vi "LoadWaveShape.vi"(8 "error in":errorcluster) -> (0 "error out":errorcluster)   [LabVIEW 2018, in "AcPwrPlugins.lvlib" / "NHRGridSim.lvclass"]
uses:
  NHRGridSim.lvclass
panel:
  in  "State":enum16{"Initialize", "Events"}(ring)
  out "XY Graph":cluster{"X":dbl, "Y":dbl}[](graph)
  out "Q4":picture
  out "Q3":picture
  out "Q2":picture
  out "Q1":picture
  out "FileName":string
  in  "Load Button":bool
  out "Data":string
  out "Qx4":dbl[](array[numeric])
  out "Qx3":dbl[](array[numeric])
  out "Qx2":dbl[](array[numeric])
  out "Qx1":dbl[](array[numeric])
  out "Quad4":dbl[](array[numeric])
  out "Quad3":dbl[](array[numeric])
  out "Quad2":dbl[](array[numeric])
  out "Quad1":dbl[](array[numeric])
  in  "Cancel Button":bool
  in  "OK Button":bool
  in  "User":enum32{"User2", "User3", "User4"}(radio)
  # "Open the file containing the Wave Shape data to be loaded into the specified NHR \"USER\" AC instrument:"
  # "Load waveform to..."
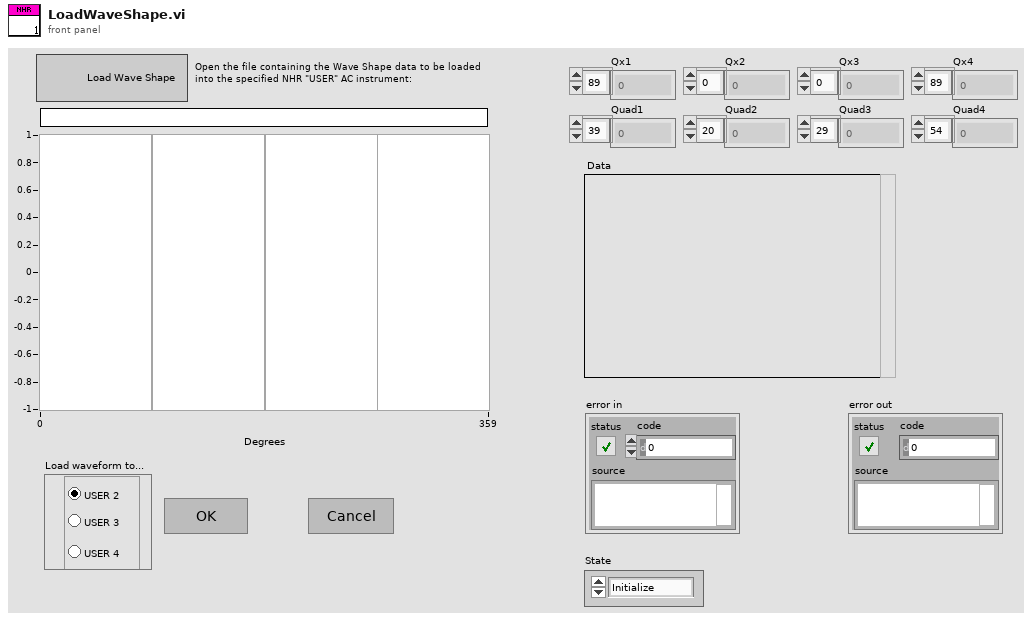
[diagram p1: front panel]
types:
  T1 = typedef "LVRectTypeDef.ctl" = cluster{"Left":i16, "Top":i16, "Right":i16, "Bottom":i16}
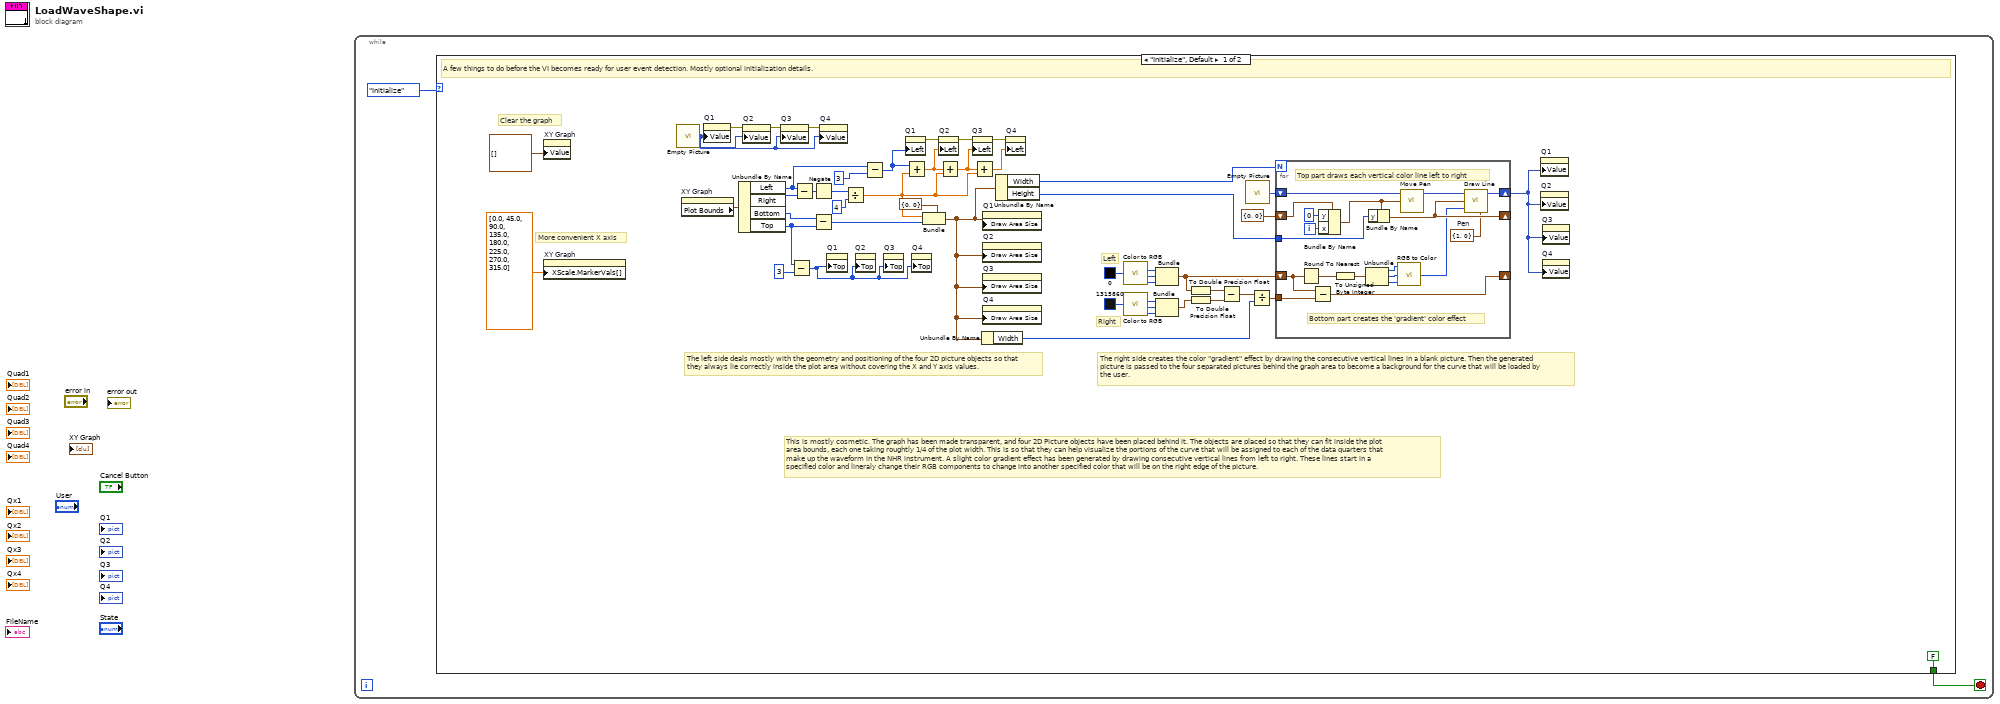
[diagram p0: block diagram]
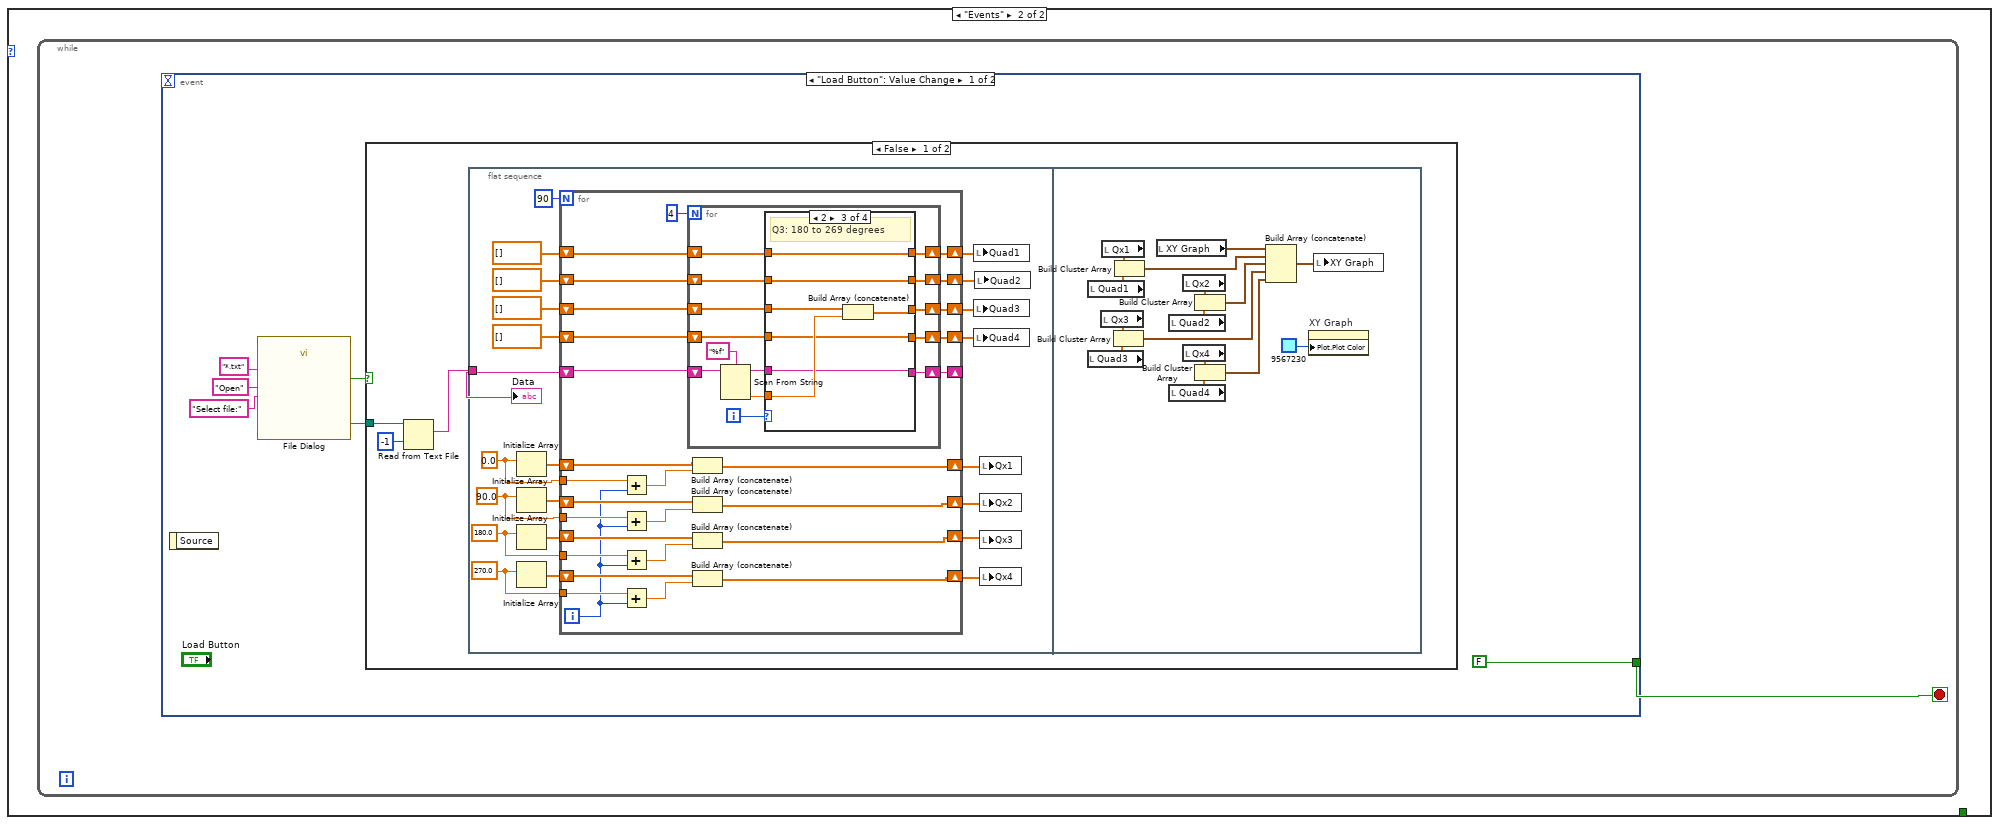
[diagram p2: hidden frame]
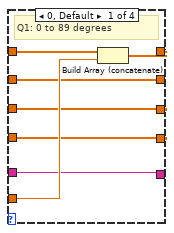
[diagram p3: hidden frame]
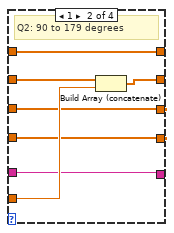
[diagram p4: hidden frame]
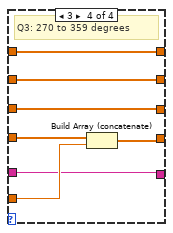
[diagram p5: hidden frame]
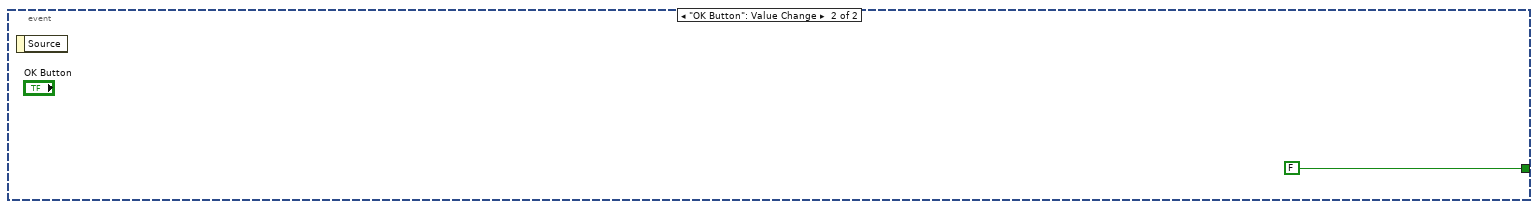
[diagram p7: hidden frame]
diagram:
  n1 = while {
    stop <- w1 stop-if-true
    n2 = case shown="\"Initialize\", Default" enum16{"Initialize", "Events"}."Initialize" ("State") {
      tunnel: [FALSE _] -> w1
      frame "Initialize", Default {
        # "The right side creates the color \"gradient\" effect by drawing the consecutive vertical lines in a blank picture. Then the generated picture is passed to the four separated pictures behind the graph area to become a background for the curve that will be loaded by the user."
        # "The left side deals mostly with the geometry and positioning of the four 2D picture objects so that they always lie correctly inside the plot area without covering the X and Y axis values."
        # "This is mostly cosmetic. The graph has been made transparent, and four 2D Picture objects have been placed behind it. The objects are placed so that they can fit inside the plot area bounds, each one taking roughtly 1/4 of the plot width. This is so that they can help visualize the portions of the curve that will be assigned to each of the data quarters that make up the waveform in the NHR instrument. A slight color gradient effect has been generated by drawing consecutive vertical lines from left to right. These lines start in a specified color and lineraly change their RGB components to change into another specified color that will be on the right edge of the picture."
        # "Right"
        # "Left"
        # "Clear the graph"
        # "More convenient X axis"
        # "A few things to do before the VI becomes ready for user event detection. Mostly optional initialization details."
        n3 = property on="XY Graph" class="XYGraph (strict)"("Value"=cluster{"element":dbl, dbl}[] [] ("array of clusters")) -> ()  [unwired: 2 in, 2 out]
        n4 = property on="XY Graph" class="XYGraph (strict)"("XScale.MarkerVals[]"=dbl[] [0.0, 45.0, 90.0, 135.0, 180.0, 225.0, 270.0, 315.0] ("X Scale.Marker Values[]")) -> ()  [unwired: 2 in, 2 out]
        n5 = call "Empty Picture"() -> ("empty picture"=w27:picture)
        n6 = property on="XY Graph" class="XYGraph (strict)"() -> ("Plot Bounds"=w28:T1)  [unwired: 2 in, 2 out]
        n7 = property on="Q1" class="Pict"("Value"=w27) -> (error out=w24:errorcluster)  [unwired: 2 in, 1 out]
        n8 = Unbundle By Name(w28) -> ("Left"=w45:i16, "Right"=w36:i16, "Bottom"=w48:i16, "Top"=w49:i16)
        n9 = property on="Q2" class="Pict"(error in=w24, "Value"=w27) -> (error out=w25:errorcluster)  [unwired: 1 in, 1 out]
        n10 = property on="Q3" class="Pict"(error in=w25, "Value"=w27) -> (error out=w26:errorcluster)  [unwired: 1 in, 1 out]
        n11 = Subtract(x=w49, y=i16 3) -> (x-y=w47:i16)
        n12 = Subtract(x=w45, y=w36) -> (x-y=w37:i16)
        n13 = Negate(x=w37) -> (-x=w38:i16)
        n14 = Subtract(x=w48, y=w49) -> (x-y=w23:i16)
        n15 = property on="Q4" class="Pict"(error in=w26, "Value"=w27) -> ()  [unwired: 1 in, 2 out]
        n16 = property on="Q1" class="Pict"("Top"=w47) -> ()  [unwired: 2 in, 2 out]
        n17 = Divide(x=w38, y=i16 4) -> (x/y=w29:dbl)
        n18 = property on="Q2" class="Pict"("Top"=w47) -> ()  [unwired: 2 in, 2 out]
        n19 = Subtract(x=w45, y=i16 3) -> (x-y=w46:i16)
        n20 = property on="Q3" class="Pict"("Top"=w47) -> ()  [unwired: 2 in, 2 out]
        n21 = property on="Q1" class="Pict"("Left"=w46) -> (error out=w32:errorcluster)  [unwired: 2 in, 1 out]
        n22 = Add(x=w46, y=w29) -> (x+y=w35:dbl)
        n23 = property on="Q4" class="Pict"("Top"=w47) -> ()  [unwired: 2 in, 2 out]
        n24 = Bundle(cluster=cluster{"Width":i32, "Height":i32} {"Width"=0, "Height"=0}, "Width"=w29, "Height"=w23) -> (w41:cluster{"Width":i32, "Height":i32})
        n25 = property on="Q2" class="Pict"(error in=w32, "Left"=w35) -> (error out=w31:errorcluster)  [unwired: 1 in, 1 out]
        n26 = Add(x=w35, y=w29) -> (x+y=w34:dbl)
        n27 = property on="Q3" class="Pict"(error in=w31, "Left"=w34) -> (error out=w30:errorcluster)  [unwired: 1 in, 1 out]
        n28 = Add(x=w34, y=w29) -> (x+y=w33:dbl)
        n29 = Unbundle By Name(w41) -> ("Width"=w40:i32)
        n30 = property on="Q1" class="Pict"("Draw Area Size"=w41) -> ()  [unwired: 2 in, 2 out]
        n31 = property on="Q2" class="Pict"("Draw Area Size"=w41) -> ()  [unwired: 2 in, 2 out]
        n32 = property on="Q3" class="Pict"("Draw Area Size"=w41) -> ()  [unwired: 2 in, 2 out]
        n33 = property on="Q4" class="Pict"("Draw Area Size"=w41) -> ()  [unwired: 2 in, 2 out]
        n34 = Unbundle By Name(w41) -> ("Width"=w42:i32, "Height"=w43:i32)
        n35 = property on="Q4" class="Pict"(error in=w30, "Left"=w33) -> ()  [unwired: 1 in, 2 out]
        n36 = call <vilib>:"Color to RGB.vi"("Color"=u32 0) -> ("R"=w11:u8, "G"=w12:u8, "B"=w13:u8)  [unwired: 1 out]
        n37 = call <vilib>:"Color to RGB.vi"("Color"=u32 1315860) -> ("R"=w16:u8, "G"=w15:u8, "B"=w14:u8)  [unwired: 1 out]
        n38 = Bundle("R"=w11, "G"=w12, "B"=w13) -> (w20:cluster{"R":u8, "G":u8, "B":u8})  [unwired: 1 in]
        n39 = Bundle("R"=w16, "G"=w15, "B"=w14) -> (w21:cluster{"R":u8, "G":u8, "B":u8})  [unwired: 1 in]
        n40 = To Double Precision Float(number=w20) -> (double precision float=w19:cluster{"R":dbl, "G":dbl, "B":dbl})
        n41 = To Double Precision Float(number=w21) -> (double precision float=w22:cluster{"R":dbl, "G":dbl, "B":dbl})
        n42 = Subtract(x=w19, y=w22) -> (x-y=w18:cluster{"R":dbl, "G":dbl, "B":dbl})
        n43 = call "Empty Picture"() -> ("empty picture"=w39:picture)
        n44 = Divide(x=w18, y=w40) -> (x/y=w17:cluster{"R":dbl, "G":dbl, "B":dbl})
        n45 = for {
          N: w42 -> [_]
          tunnel: w43 -> [w66]
          shift-right: [w64] -> w44
          shift-left: w39 -> [w70]
          shift-right: [w63] -> _
          shift-left: cluster{"x":i16, "y":i16} {"x"=0, "y"=0} ("new position") -> [w67]
          tunnel: w17 -> [w61]
          shift-right: [w60] -> _
          shift-left: w20 -> [w56]
          i -> [w59]
          w54 = cluster{"x":u16, "y":u32} {"x"=1, "y"=0}  # Pen
          # "Bottom part creates the 'gradient' color effect"
          # "Top part draws each vertical color line left to right"
          n46 = Round To Nearest(number=w56) -> (nearest integer value=w55:cluster{"R":dbl, "G":dbl, "B":dbl})
          n47 = Subtract(x=w56, y=w61) -> (x-y=w60:cluster{"R":dbl, "G":dbl, "B":dbl})
          n48 = Bundle By Name(cluster=w67, "y"=i16 0, "x"=w59) -> (w65:cluster{"x":i16, "y":i16})
          n49 = To Unsigned Byte Integer(number=w55) -> (unsigned 8bit integer=w58:cluster{"R":u8, "G":u8, "B":u8})
          n50 = Unbundle(w58) -> ("R"=w52:u8, "G"=w53:u8, "B"=w57:u8)
          n51 = Bundle By Name(cluster=w65, "y"=w66) -> (w63:cluster{"x":i16, "y":i16})
          n52 = call <vilib>:"RGB to Color.vi"("B"=w57, "G"=w53, "R"=w52) -> ("Color"=w62:u32)
          n53 = call <vilib>:"Move Pen.vi"("new position"=w65, "picture"=w70) -> ("new picture"=w69:picture)  [unwired: 3 in]
          n54 = call <vilib>:"Draw Line.vi"("picture"=w69, "end point"=w63, "color(black)"=w62, "pen"=w54) -> ("new picture"=w64:picture)  [unwired: 5 in]
        }
        n55 = property on="Q1" class="Pict"("Value"=w44) -> ()  [unwired: 2 in, 2 out]
        n56 = property on="Q2" class="Pict"("Value"=w44) -> ()  [unwired: 2 in, 2 out]
        n57 = property on="Q3" class="Pict"("Value"=w44) -> ()  [unwired: 2 in, 2 out]
        n58 = property on="Q4" class="Pict"("Value"=w44) -> ()  [unwired: 2 in, 2 out]
      }
      frame "Events" {
        n59 = while {
          stop <- w71 stop-if-true
          n60 = event shown="[0] \"Load Button\": Value Change" {
            selector: _ -> [_ _]
            dyn-events: _ -> [_ _]
            timeout: _ -> [_ _]
            tunnel: [FALSE FALSE] -> w71
            event "Load Button": Value Change {
              n61 = event-data() -> ()  [unwired: 1 in, 1 out]
              n62 = call "File Dialog"("prompt"="Select file:", "button label"="Open", "pattern (all files)"="*.txt") -> ("selected path"=w72:path, "cancelled"=w73:bool)  [unwired: 9 in, 2 out]
              n63 = case shown="False" w73 {
                tunnel: w72 -> [w80 _]
                frame False {
                  n64 = Read from Text File(file (use dialog)=w80, count=-1) -> (text=w78:string)  [unwired: 2 in, 3 out]
                  n65 = flat-sequence {
                    tunnel: w78 -> [w81]
                    frame #0 {
                      w90 = 270.0 ("element")
                      w89 = 180.0 ("element")
                      w88 = 90.0 ("element")
                      w87 = 0.0 ("element")
                      n66 = Initialize Array(w87) -> (w102:dbl[])  [unwired: 1 in]
                      n67 = Initialize Array(w88) -> (w101:dbl[])  [unwired: 1 in]
                      n68 = Initialize Array(w89) -> (w100:dbl[])  [unwired: 1 in]
                      n69 = Initialize Array(w90) -> (w99:dbl[])  [unwired: 1 in]
                      n70 = for {
                        N: 90 -> [_]
                        shift-right: [w126] -> w98
                        shift-left: dbl[] [] -> [w129]
                        shift-right: [w125] -> w97
                        shift-left: dbl[] [] -> [w122]
                        shift-right: [w124] -> w96
                        shift-left: dbl[] [] -> [w128]
                        shift-right: [w123] -> w95
                        shift-left: dbl[] [] -> [w127]
                        tunnel: w87 -> [w120]
                        tunnel: w88 -> [w118]
                        tunnel: w89 -> [w113]
                        shift-right: [w112] -> w91
                        shift-left: w102 -> [w119]
                        shift-right: [w111] -> w92
                        shift-left: w101 -> [w117]
                        shift-right: [w110] -> w93
                        shift-left: w100 -> [w115]
                        shift-right: [w108] -> w94
                        shift-left: w99 -> [w109]
                        tunnel: w90 -> [w107]
                        shift-right: [w103] -> _
                        shift-left: w81 -> [w104]
                        i -> [w106]
                        n71 = Add(x=w120, y=w106) -> (x+y=w121:dbl)
                        n72 = Add(x=w118, y=w106) -> (x+y=w116:dbl)
                        n73 = Add(x=w113, y=w106) -> (x+y=w114:dbl)
                        n74 = Add(x=w107, y=w106) -> (x+y=w105:dbl)
                        n75 = for {
                          N: 4 -> [_]
                          shift-right: [w142] -> w126
                          shift-left: w129 -> [w143]
                          shift-right: [w141] -> w125
                          shift-left: w122 -> [w136]
                          shift-right: [w139] -> w124
                          shift-left: w128 -> [w140]
                          shift-right: [w137] -> w123
                          shift-left: w127 -> [w138]
                          shift-right: [w131] -> w103
                          shift-left: w104 -> [w133]
                          i -> [w144]
                          n76 = Scan From String(format string="%f", input string=w133) -> (remaining string=w132:string, output 1=w134:dbl)  [unwired: 3 in, 2 out]
                          n77 = case shown="2" w144 {
                            tunnel: w143 -> [w151 w153 w163 w171]
                            tunnel: w134 -> [w150 w158 w165 w172]
                            tunnel: [w149 w153 w163 w171] -> w142
                            tunnel: w136 -> [w148 w155 w160 w170]
                            tunnel: [w148 w154 w160 w170] -> w141
                            tunnel: w140 -> [w147 w157 w162 w167]
                            tunnel: [w147 w157 w161 w167] -> w139
                            tunnel: w138 -> [w146 w156 w164 w169]
                            tunnel: [w146 w156 w164 w168] -> w137
                            tunnel: [w145 w152 w159 w166] -> w131
                            tunnel: w132 -> [w145 w152 w159 w166]
                            frame 0, Default {
                              # "Q1: 0 to 89 degrees"
                              n78 = Build Array (concatenate)(w151, w150) -> (w149:dbl[])
                            }
                            frame 1 {
                              # "Q2: 90 to 179 degrees"
                              n79 = Build Array (concatenate)(w155, w158) -> (w154:dbl[])
                            }
                            frame 2 {
                              # "Q3: 180 to 269 degrees"
                              n80 = Build Array (concatenate)(w162, w165) -> (w161:dbl[])
                            }
                            frame 3 {
                              # "Q3: 270 to 359 degrees"
                              n81 = Build Array (concatenate)(w169, w172) -> (w168:dbl[])
                            }
                          }
                        }
                        n82 = Build Array (concatenate)(w119, w121) -> (w112:dbl[])
                        n83 = Build Array (concatenate)(w117, w116) -> (w111:dbl[])
                        n84 = Build Array (concatenate)(w115, w114) -> (w110:dbl[])
                        n85 = Build Array (concatenate)(w109, w105) -> (w108:dbl[])
                      }
                      n86 = local write "Quad1"(w98) -> ()
                      n87 = local write "Quad3"(w96) -> ()
                      n88 = local write "Quad4"(w95) -> ()
                      n89 = local write "Quad2"(w97) -> ()
                      n90 = local write "Qx1"(w91) -> ()
                      n91 = local write "Qx2"(w92) -> ()
                      n92 = local write "Qx3"(w93) -> ()
                      n93 = local write "Qx4"(w94) -> ()
                      "Data" <- w81
                    }
                    frame #1 {
                      n94 = local read "Quad3"() -> (w181:dbl[])
                      n95 = local read "Quad1"() -> (w186:dbl[])
                      n96 = local read "Qx3"() -> (w182:dbl[])
                      n97 = local read "Qx1"() -> (w187:dbl[])
                      n98 = Build Cluster Array(w182, w181) -> (w177:cluster{"element":dbl, dbl}[])
                      n99 = Build Cluster Array(w187, w186) -> (w185:cluster{"element":dbl, dbl}[])
                      n100 = local read "XY Graph"() -> (w175:cluster{"X":dbl, "Y":dbl}[])
                      n101 = local read "Quad2"() -> (w184:dbl[])
                      n102 = local read "Quad4"() -> (w180:dbl[])
                      n103 = local read "Qx2"() -> (w183:dbl[])
                      n104 = local read "Qx4"() -> (w179:dbl[])
                      n105 = Build Cluster Array(w183, w184) -> (w178:cluster{"element":dbl, dbl}[])
                      n106 = Build Cluster Array(w179, w180) -> (w176:cluster{"element":dbl, dbl}[])
                      n107 = Build Array (concatenate)(w175, w185, w178, w177, w176) -> (w174:cluster{"element":dbl, "Y":dbl}[])
                      n108 = property on="XY Graph" class="XYGraph (strict)"("Plot.Plot Color"=u32 9567230) -> ()  [unwired: 2 in, 2 out]
                      n109 = local write "XY Graph"(w174) -> ()
                    }
                  }
                }
                frame True {
                }
              }
            }
            event "OK Button": Value Change {
              n110 = event-data() -> ()  [unwired: 1 in, 1 out]
            }
          }
        }
      }
    }
  }
